vi "abc.vi"(11 "Platter in":T1 format="%032b") -> (0 "C":i32, 1 "B":i32, 2 "A":i32)   [LabVIEW 2020]
uses:
  Platter.ctl
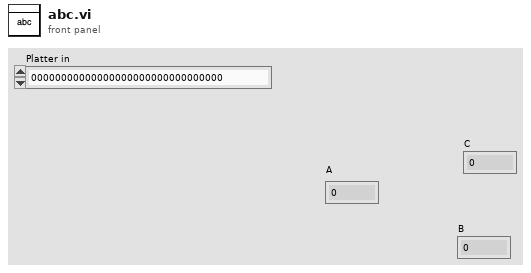
[diagram p1: front panel]
types:
  T1 = typedef "Platter.ctl" = u32
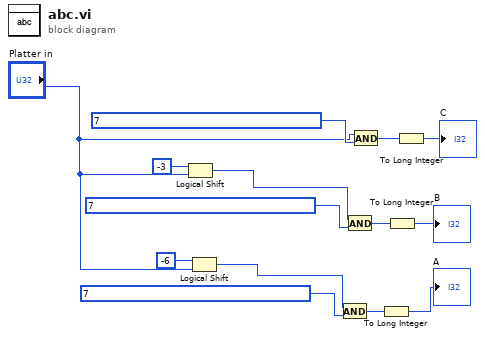
[diagram p0: block diagram]
diagram:
  n1 = Logical Shift(y=i16 -3, x="Platter in") -> (x << y=w7:T1)
  n2 = Logical Shift(y=i16 -6, x="Platter in") -> (x << y=w5:T1)
  n3 = And(x=w5, y=T1 7) -> (x .and. y?=w4:T1)
  n4 = And(x=w7, y=T1 7) -> (x .and. y?=w9:T1)
  n5 = And(x="Platter in", y=T1 7) -> (x .and. y?=w10:T1)
  n6 = To Long Integer(number=w4) -> (32bit integer=→"A":i32)
  n7 = To Long Integer(number=w9) -> (32bit integer=→"B":i32)
  n8 = To Long Integer(number=w10) -> (32bit integer=→"C":i32)
